vi "transfer.vi"(0 "输入":string) -> (1 "数值":u8, 2 "布尔":bool, 3 "输出":string)   [LabVIEW 2014]
panel:
  out "无符号字节数组":u8[](array[numeric])
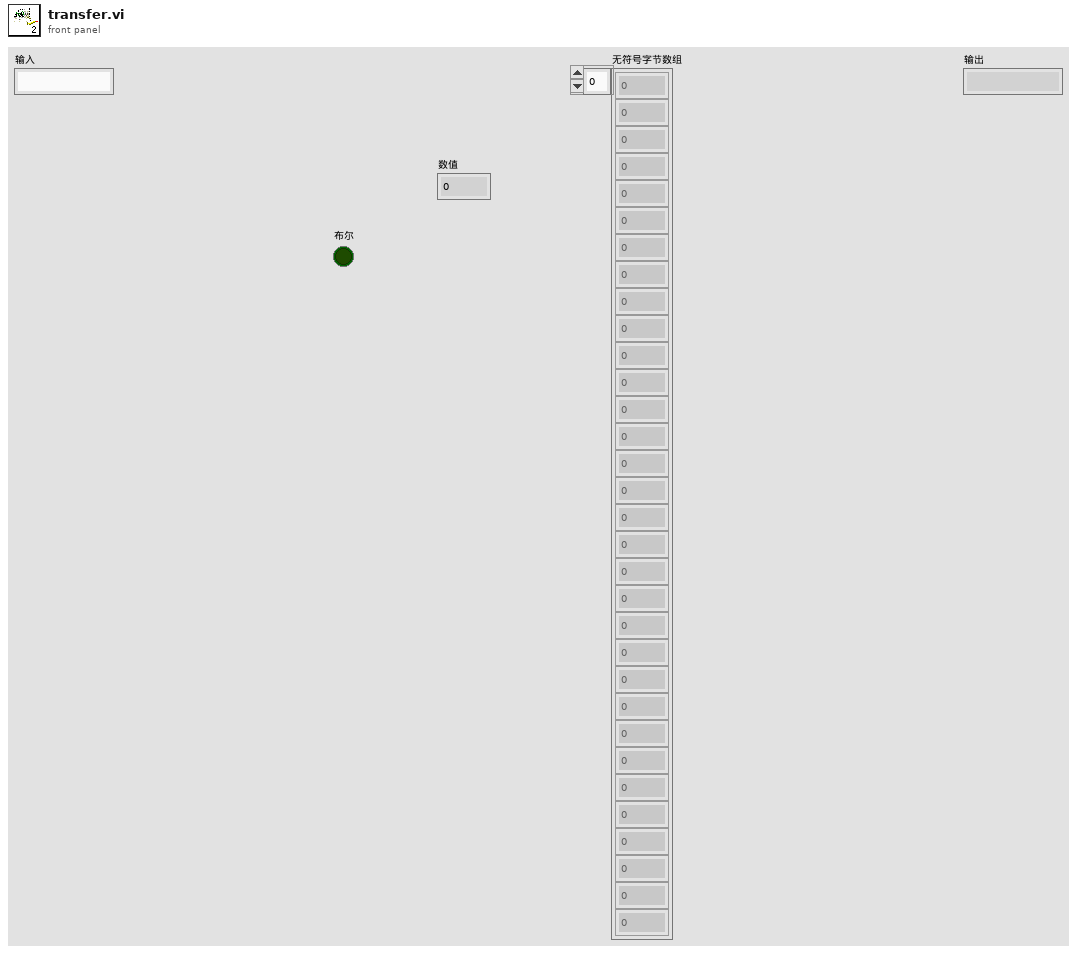
[diagram p1: front panel]
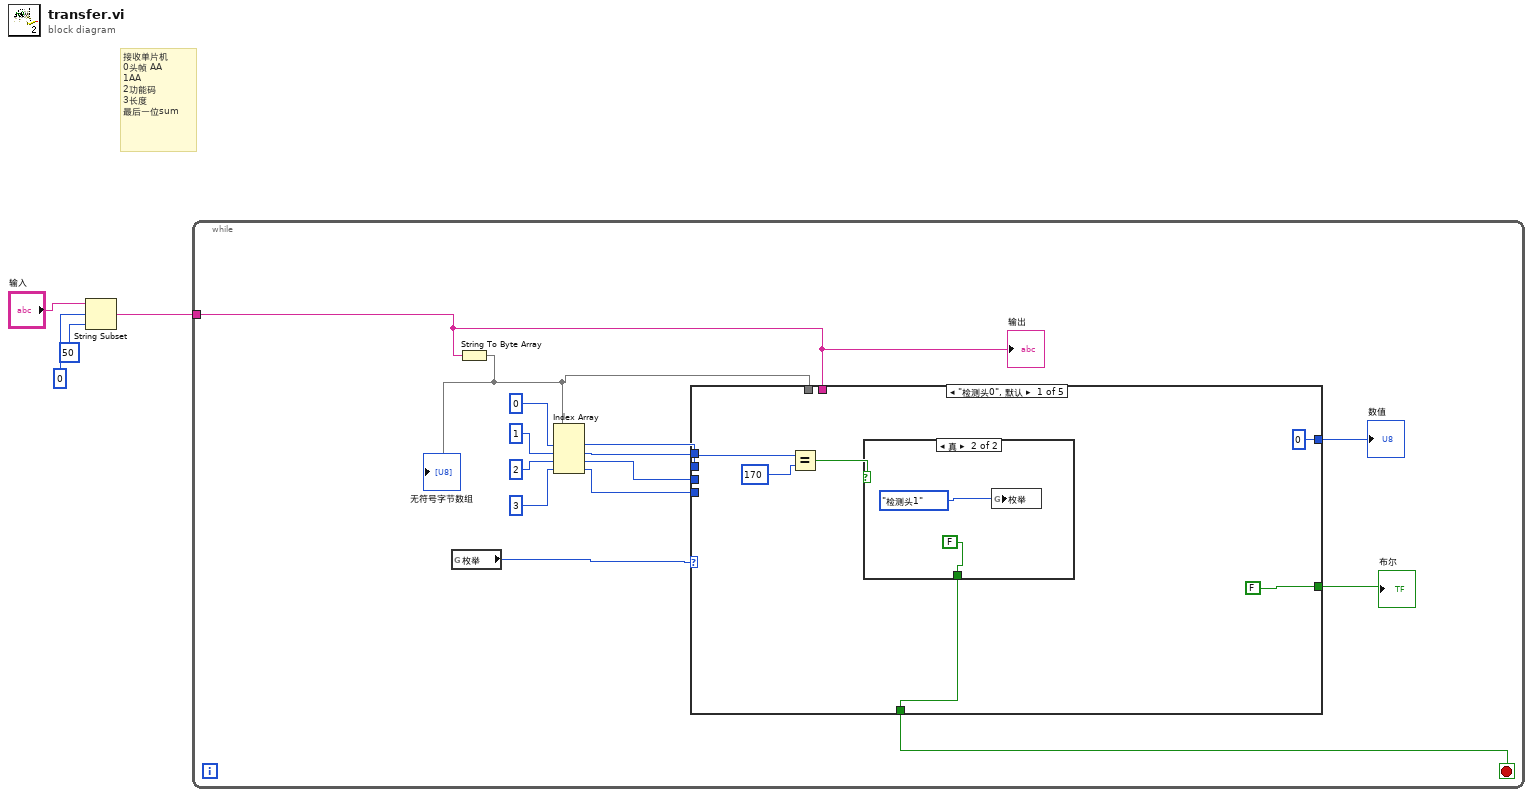
[diagram p0: block diagram]
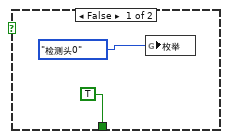
[diagram p2: hidden frame]
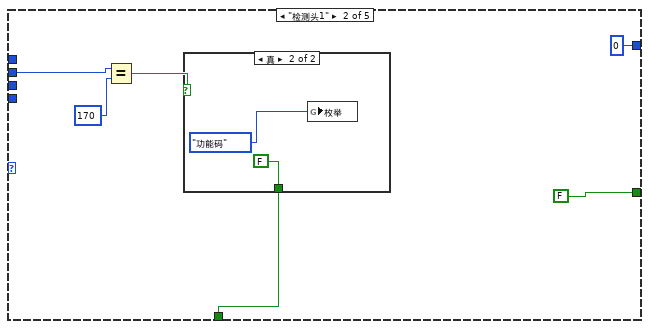
[diagram p3: hidden frame]
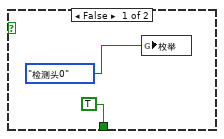
[diagram p4: hidden frame]
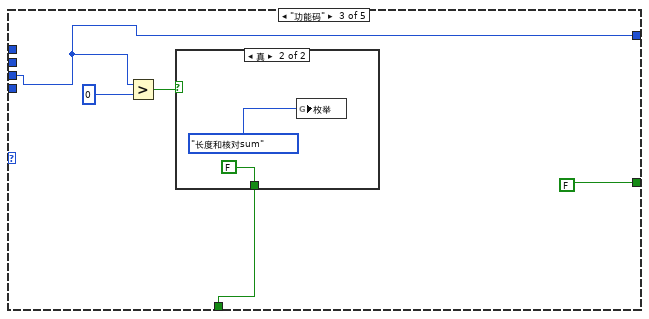
[diagram p5: hidden frame]
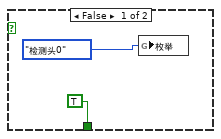
[diagram p6: hidden frame]
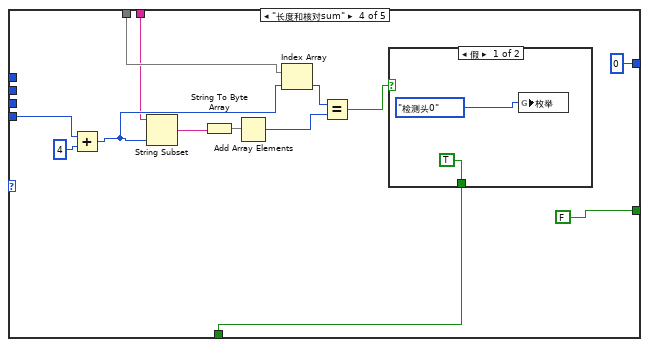
[diagram p7: hidden frame]
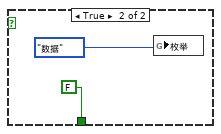
[diagram p8: hidden frame]
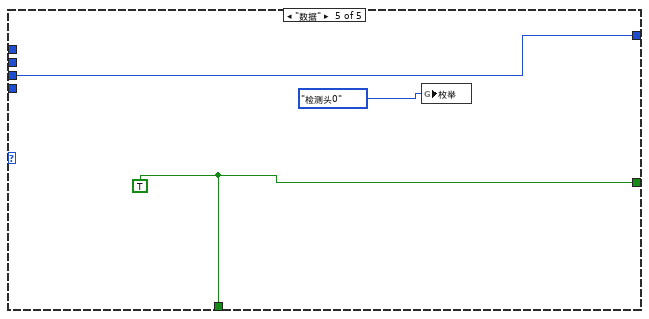
[diagram p9: hidden frame]
diagram:
  # "接收单片机\n0头帧 AA \n1AA\n2功能码\n3长度\n最后一位sum"
  n1 = String Subset(string="输入", offset (0)=0 ("长度（剩余）"), length (rest)=50 ("长度（剩余）")) -> (substring=w3:string)
  n2 = while {
    tunnel: w3 -> [w5]
    stop <- w6 stop-if-true
    n3 = global read "全局变量.vi" "枚举"() -> (w9:enum16{"检测头0", "检测头1", "功能码", "长度和核对sum", "数据"})
    n4 = String To Byte Array(string=w5) -> (unsigned byte array=w10:u8[])
    "无符号字节数组" <- w10
    n5 = Index Array(array=w10, index #1=0 ("长度（剩余）"), index #2=1 ("长度（剩余）"), index #3=2 ("索引"), index #4=3 ("索引")) -> (element #1=w14:u8, element #2=w13:u8, element #3=w12:u8, element #4=w11:u8)
    n6 = case shown="\"检测头0\", 默认" w9 {
      tunnel: w14 -> [w22 _ _ _ _]
      tunnel: w13 -> [_ w32 _ _ _]
      tunnel: w12 -> [_ _ w40 _ w65]
      tunnel: w11 -> [_ _ _ w59 _]
      tunnel: w10 -> [_ _ _ w56 _]
      tunnel: w5 -> [_ _ _ w51 _]
      tunnel: [FALSE ("布尔") FALSE ("布尔") FALSE ("布尔") FALSE ("布尔") w66] -> w8
      tunnel: [u8 0 u8 0 w40 u8 0 w65] -> w7
      tunnel: [w19 w29 w39 w48 w66] -> w6
      frame "检测头0", Default {
        n7 = Equal?(x=w22, y=170 ("长度（剩余）")) -> (x = y?=w23:bool)
        n8 = case shown="真" w23 {
          tunnel: [TRUE FALSE ("布尔")] -> w19
          frame False {
            n9 = global write "全局变量.vi" "枚举"(enum16{"检测头0", "检测头1", "功能码", "长度和核对sum", "数据"}."检测头0" ("枚举")) -> ()
          }
          frame True {
            n10 = global write "全局变量.vi" "枚举"(enum16{"检测头0", "检测头1", "功能码", "长度和核对sum", "数据"}."检测头1" ("枚举")) -> ()
          }
        }
      }
      frame "检测头1" {
        n11 = Equal?(x=w32, y=170 ("长度（剩余）")) -> (x = y?=w33:bool)
        n12 = case shown="真" w33 {
          tunnel: [TRUE FALSE ("布尔")] -> w29
          frame False {
            n13 = global write "全局变量.vi" "枚举"(enum16{"检测头0", "检测头1", "功能码", "长度和核对sum", "数据"}."检测头0" ("枚举")) -> ()
          }
          frame True {
            n14 = global write "全局变量.vi" "枚举"(enum16{"检测头0", "检测头1", "功能码", "长度和核对sum", "数据"}."功能码" ("枚举")) -> ()
          }
        }
      }
      frame "功能码" {
        n15 = Greater?(x=w40, y=u8 0) -> (0:w42:bool)
        n16 = case shown="真" w42 {
          tunnel: [TRUE FALSE ("布尔")] -> w39
          frame False {
            n17 = global write "全局变量.vi" "枚举"(enum16{"检测头0", "检测头1", "功能码", "长度和核对sum", "数据"}."检测头0" ("枚举")) -> ()
          }
          frame True {
            n18 = global write "全局变量.vi" "枚举"(enum16{"检测头0", "检测头1", "功能码", "长度和核对sum", "数据"}."长度和核对sum" ("枚举")) -> ()
          }
        }
      }
      frame "长度和核对sum" {
        n19 = Add(x=w59, y=u8 4) -> (x+y=w55:u8)
        n20 = String Subset(string=w51, length (rest)=w55) -> (substring=w58:string)  [unwired: 1 in]
        n21 = String To Byte Array(string=w58) -> (unsigned byte array=w57:u8[])
        n22 = Add Array Elements(numeric array=w57) -> (sum=w53:u8)
        n23 = Index Array(array=w56, index=w55) -> (element=w54:u8)
        n24 = Equal?(x=w54, y=w53) -> (x = y?=w52:bool)
        n25 = case shown="假" w52 {
          tunnel: [TRUE FALSE ("布尔")] -> w48
          frame False {
            n26 = global write "全局变量.vi" "枚举"(enum16{"检测头0", "检测头1", "功能码", "长度和核对sum", "数据"}."检测头0" ("枚举")) -> ()
          }
          frame True {
            n27 = global write "全局变量.vi" "枚举"(enum16{"检测头0", "检测头1", "功能码", "长度和核对sum", "数据"}."数据" ("枚举")) -> ()
          }
        }
      }
      frame "数据" {
        w66 = TRUE ("布尔")
        n28 = global write "全局变量.vi" "枚举"(enum16{"检测头0", "检测头1", "功能码", "长度和核对sum", "数据"}."检测头0" ("枚举")) -> ()
      }
    }
    "布尔" <- w8
    "数值" <- w7
    "输出" <- w5
  }
